vi "Read Tiff File.vi"(5 "Create Flattened Images (24 Bit only)":bool, 8 "error in (no error)":errorcluster, 11 "Path":path) -> (0 "error out":errorcluster, 1 "Flattened Images":T1[](array[typedef]), 2 "Pages":cluster{"Image Data":variant, "Details":T2}[](array[cluster]) {"Details"."PhotometricInterpretation" items=["MIN IS WHITE"=0, "MIN IS BLACK"=1, "RGB"=2, "PALETTE"=3, "MASK"=4, "SEPARATED"=5, "YCBCR"=6, "CIE LAB"=8, "ICC LAB"=9, "ITU LAB"=10, "LOGL"=32844, "LOGLUV"=32845, "CFA"=32803, "LinearRaw"=34892, "DEPTH"=51177]}, 3 "path":path)   [LabVIEW 2020, in "LV Tiff.lvlib" / "TIFF Reader.lvclass"]
uses:
  TIFF Reader.lvclass
  _Helpers/Tiff Page Details.ctl
  TIFF Reader.lvclass/TIFF Reader.ctl
  LV Tiff.lvlib
  <vilib>/picture/picture.llb/imagedata.ctl
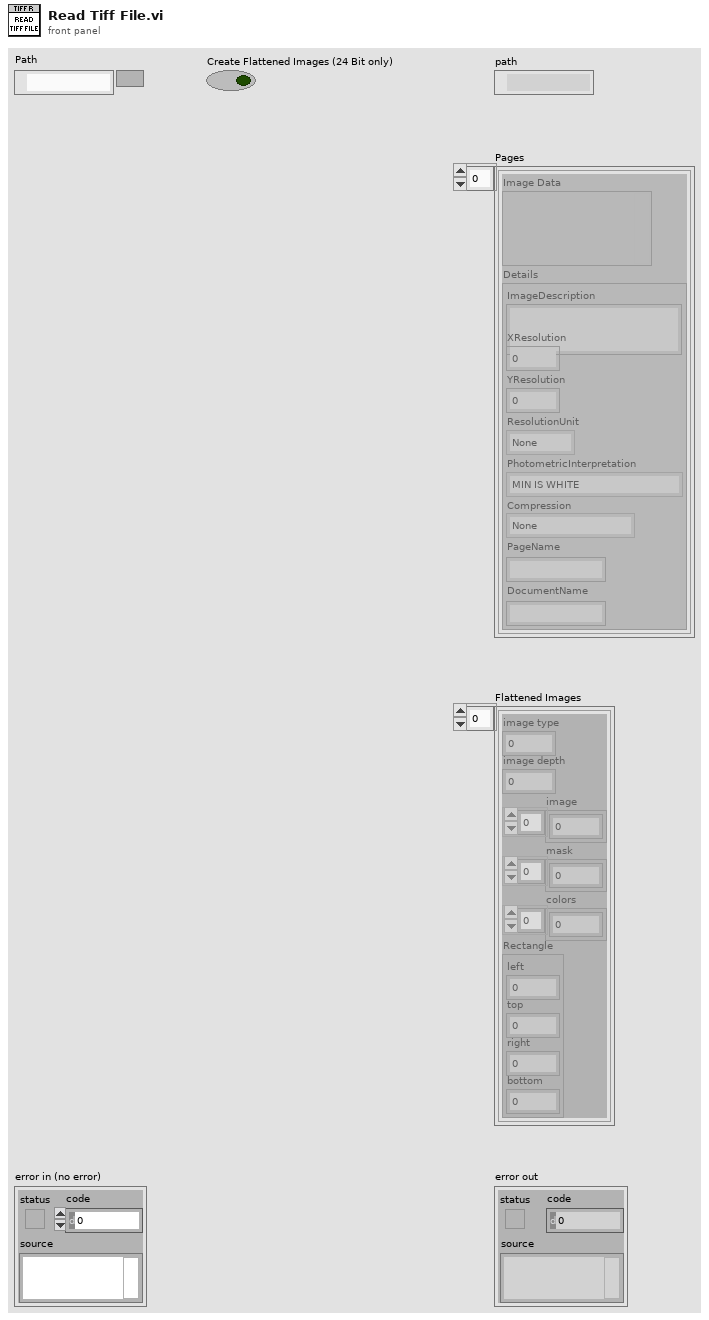
[diagram p1: front panel]
types:
  T1 = typedef "imagedata.ctl" = cluster{"image type":i32, "image depth":i32, "image":u8[], "mask":u8[], "colors":u32[], "Rectangle":cluster{"left":i16, "top":i16, "right":i16, "bottom":i16}}
  T2 = typedef "LV Tiff.lvlib/Tiff Page Details.ctl" = cluster{"ImageDescription":string, "XResolution":dbl, "YResolution":dbl, "ResolutionUnit":enum16{"None", "Inch", "Centimeter"}, "PhotometricInterpretation":u16, "Compression":enum16{"None", "Deflate", "JPEG"}, "PageName":string, "DocumentName":string}
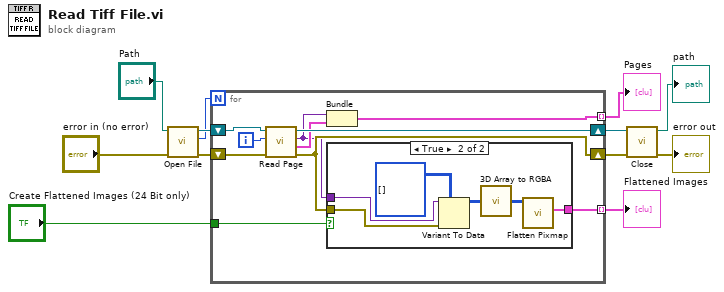
[diagram p0: block diagram]
diagram:
  n1 = call "Open File.vi"("error in (no error)"="error in (no error)", "Path"="Path") -> ("error out"=w10:errorcluster, "N Pages"=w5:i32, "TIFF Reader.lvclass"=w9:refnum<class "TIFF Reader.lvclass">)  [unwired: 7 in]
  n2 = for {
    N: w5 -> [_]
    shift-right: [w16] -> w7
    shift-left: w10 -> [w22]
    shift-right: [w20] -> w8
    shift-left: w9 -> [w21]
    tunnel: [w17] -> w4 mode=indexing
    tunnel: [w14] -> w2 mode=indexing
    tunnel: "Create Flattened Images (24 Bit only)" -> [w13]
    i -> [w19]
    n3 = call "Read Page.vi"("error in (no error)"=w22, "index"=w19, "TIFF Reader in"=w21) -> ("error out"=w16:errorcluster, "Details"=w18:T2, "Image Data"=w15:variant, "TIFF Reader out"=w20:refnum<class "TIFF Reader.lvclass">)  [unwired: 4 in, 1 out]
    n4 = Bundle("Image Data"=w15, "Details"=w18) -> (w17:cluster{"Image Data":variant, "Details":T2})  [unwired: 1 in]
    n5 = case shown="True" w13 {
      tunnel: w16 -> [_ w28]
      tunnel: w15 -> [_ w27]
      tunnel: [_ w23] -> w14
      frame False {
      }
      frame True {
        n6 = Variant To Data(error in=w28, type=u8[][][] [], Variant=w27) -> (data=w25:u8[][][])  [unwired: 1 out]
        n7 = call "3D Array to RGBA.vi"("3D Array"=w25) -> ("RGBA"=w24:u32[][])
        n8 = call <vilib>:"Flatten Pixmap.vi"("24-bit pixmap"=w24) -> ("image data"=w23:T1)  [unwired: 10 in]
      }
    }
  }
  "Pages" <- w4
  "Flattened Images" <- w2
  n9 = call "Close.vi"("error in (no error)"=w7, "TIFF Reader in"=w8) -> ("error out"=→"error out":errorcluster, "path"=→"path":path)  [unwired: 8 in]
